vi "Power Down 4137.vi"(8 "error in (no error)":errorcluster, 11 "Semiconductor Module Context":T1) -> (0 "error out":errorcluster)   [LabVIEW 2019]
uses:
  <vilib>/NI_TestStand_SemiconductorModule/NI_TestStand_Semiconductor_Module.lvlibp/PinMap/General/SemiconductorModuleContext.ctl
  <vilib>/NI_TestStand_SemiconductorModule/NI_TestStand_Semiconductor_Module.lvlibp
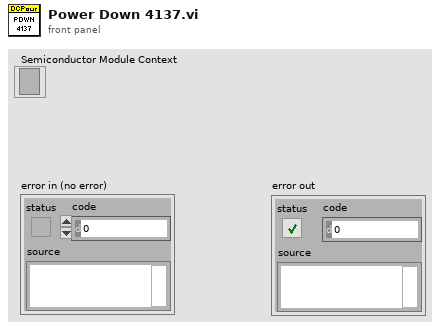
[diagram p1: front panel]
types:
  T1 = typedef "NI_TestStand_Semiconductor_Module.lvlibp/SemiconductorModuleContext.ctl" = refnum<k7>
  T2 = typedef "TSM SSC DCPower.ctl" = cluster{"Pin Query Context":refnum<class "MultiplePinMultipleSessionQueryContext.lvclass">, "SSC":T3[], "Site Numbers":i32[], "Pins":T4[], "Pins Expanded":T6[]}
  T3 = typedef "SSC DCPower.ctl" = cluster{"Session":refnum<k15>, "Chan":string, "Channel List":string}
  T4 = typedef "TSM Pin Information.ctl" = cluster{"Pin":tag, "Type":T5, "Count":i32}
  T5 = typedef "TSM Pin Type Identifier.ctl" = enum8{"DUT Pin", "System Pin", "Pin Group", "Not Determined"}
  T6 = typedef "TSM Expanded Pin Information.ctl" = cluster{"Pin":tag, "Type":T5, "Index":i32}
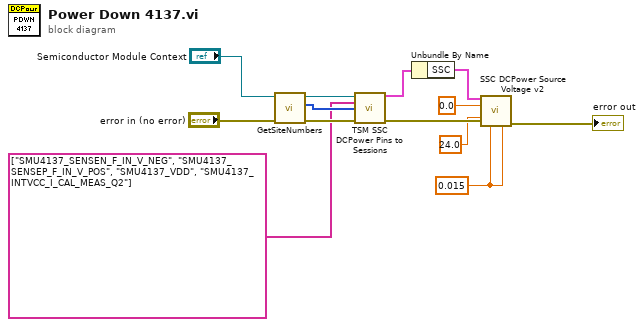
[diagram p0: block diagram]
diagram:
  w3 = 0.015 ("Current Limit, A")
  n1 = call <vilib>:"GetSiteNumbers.vi"("error in (no error)"="error in (no error)", "Semiconductor Module Context"="Semiconductor Module Context") -> ("error out"=w13:errorcluster, "Site Numbers"=w11:i32[], "Semiconductor Module Context Out"=w12:T1)  [unwired: 6 in, 1 out]
  n2 = call "TSM SSC DCPower Pins to Sessions.vi"("TSM context"=w12, "Pins"=tag[] ["SMU4137_SENSEN_F_IN_V_NEG", "SMU4137_SENSEP_F_IN_V_POS", "SMU4137_VDD", "SMU4137_INTVCC_I_CAL_MEAS_Q2"], "Site Numbers"=w11, "error in"=w13) -> ("DCPower TSM Out"=w7:T2, "error out"=w8:errorcluster)  [unwired: 10 in]
  n3 = Unbundle By Name(w7) -> ("SSC"=w6:T3[])
  n4 = call "SSC DCPower Source Voltage v2.vi"("DCPower SSC in"=w6, "Voltage Level, V"=0.0, "Voltage Level Range (V)"=24.0, "error in"=w8, "Current Limit, A"=w3, "Current Limit Range (A)"=w3) -> ("error out"=→"error out":errorcluster)  [unwired: 8 in, 1 out]
